vi "Init.vi"(8 "error in (no error)":errorcluster, 10 "Channel":i16, 11 "TrialBasedExperiment in":refnum<class "WhiteNoiseOrientationDetection.lvclass">) -> (0 "error out":errorcluster, 3 "TrialBasedExperiment out":refnum<class "WhiteNoiseOrientationDetection.lvclass">)   [LabVIEW 2014, in "WhiteNoiseOrientationDetection.lvclass"]
uses:
  WhiteNoiseOrientationDetection.lvclass
  WhiteNoiseOrientationDetection.lvclass/WhiteNoiseOrientationDetection.ctl
  Trial Based Experiment Statechart/MatlabExperiment/MatlabExperiment.lvclass
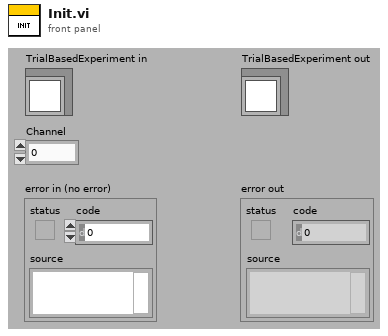
[diagram p1: front panel]
types:
  T1 = cluster{"Intertrial":dbl, "AcquireFixation":dbl, "HoldFixation":dbl, "DelayPeriod":dbl, "ResponsePeriod":dbl}
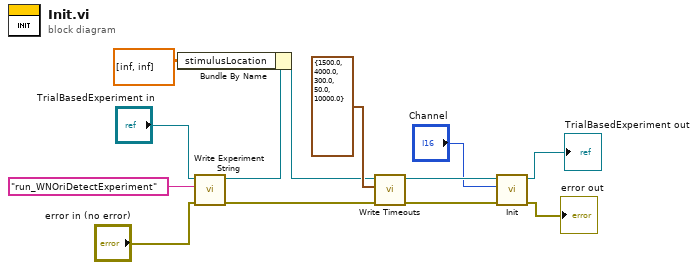
[diagram p0: block diagram]
diagram:
  n1 = call-dynamic "Write Experiment String.vi"("error in (no error)"="error in (no error)", "Experiment String"="run_WNOriDetectExperiment", "TrialBasedExperiment in"="TrialBasedExperiment in") -> ("error out"=w12:errorcluster, "TrialBasedExperiment out"=w2:refnum<class "WhiteNoiseOrientationDetection.lvclass">)  [unwired: 7 in]
  n2 = Bundle By Name(cluster=w2, "stimulusLocation"=dbl[][] [[inf, inf]]) -> (w1:refnum<class "WhiteNoiseOrientationDetection.lvclass">)
  n3 = call-dynamic "Write Timeouts.vi"("error in (no error)"=w12, "Timeouts"=T1 {"Intertrial"=1500.0, "AcquireFixation"=4000.0, "HoldFixation"=300.0, "DelayPeriod"=50.0, "ResponsePeriod"=10000.0}, "TrialBasedExperiment in"=w1) -> ("error out"=w11:errorcluster, "TrialBasedExperiment out"=w10:refnum<class "WhiteNoiseOrientationDetection.lvclass">)  [unwired: 7 in]
  n4 = call-parent "Init.vi"("error in (no error)"=w11, "Channel"="Channel", "TrialBasedExperiment in"=w10) -> ("error out"=→"error out":errorcluster, "TrialBasedExperiment out"=→"TrialBasedExperiment out":refnum<class "WhiteNoiseOrientationDetection.lvclass">)  [unwired: 7 in]
